vi "UnitTestSimulation.vi"(8 "error in (no error)":errorcluster) -> (0 "error out":errorcluster, 1 "LowerLimit":dbl[](array[numeric]), 2 "UpperLimit":dbl[](array[numeric]), 3 "Limit Testing":dbl[][](graph))   [LabVIEW 2021]
uses:
  <vilib>/measure/NI_MABase.lvlib
panel:
  in  "Signal":dbl[](array[numeric])=[1.1, 1.1, -0.9, -0.9, 1.1, 1.1, -0.9, -0.9, 1.1, 1.1, -0.9]
  out "Waveform":dbl[](array[numeric])
  in  "Upper Limit Y values":dbl[](array[numeric])=[1.1, 1.1, -0.9, -0.9, 1.1, 1.1, -0.9, -0.9, 1.1, 1.1, -0.9]
  in  "Lower Limit Y values":dbl[](array[numeric])=[0.9, 0.9, -1.1, -1.1, 0.9, 0.9, -1.1, -1.1, 0.9, 0.9, -1.1]
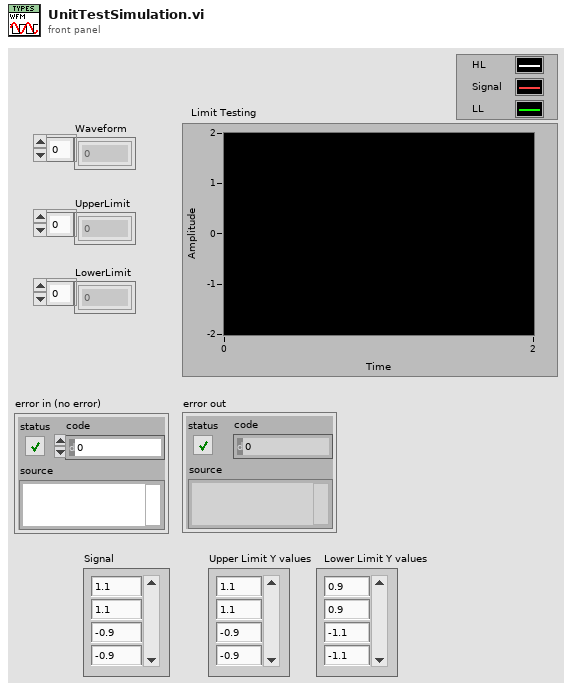
[diagram p1: front panel]
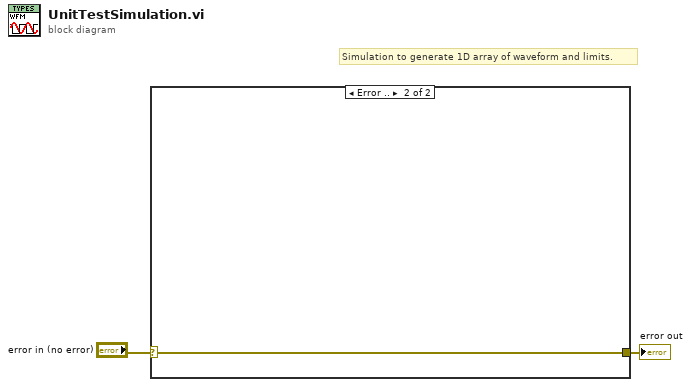
[diagram p0: block diagram]
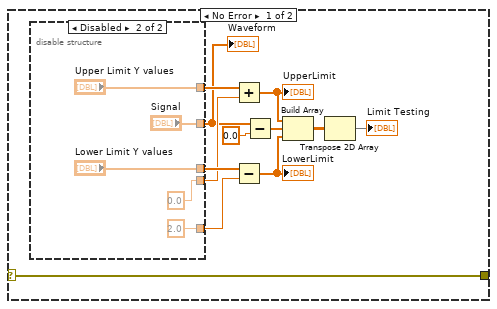
[diagram p2: hidden frame]
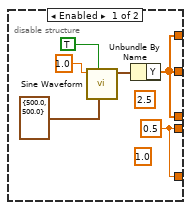
[diagram p3: hidden frame]
diagram:
  # "Simulation to generate 1D array of waveform and limits."
  n1 = case shown="Error .." "error in (no error)" {
    selector: "error in (no error)" -> [w3 w26]
    tunnel: [w3 w26] -> w1
    frame No Error {
      n2 = disable-structure shown="Disabled" {
        disable-tunnel: [w16 "Signal"] -> w6
        disable-tunnel: [w16 "Upper Limit Y values"] -> w10
        disable-tunnel: [w16 "Lower Limit Y values"] -> w9
        disable-tunnel: [w15 0.0] -> w8
        disable-tunnel: [w15 2.0] -> w7
        frame Enabled {
          (unwired) 1.0
          w15 = 0.5
          (unwired) 2.5 ("frequency")
          n3 = call <vilib>:"Sine Waveform.vi"("sampling info"=cluster{"Fs":dbl, "#s":dbl} {"Fs"=500.0, "#s"=500.0}, "reset signal"=TRUE, "frequency"=1.0) -> ("signal out"=w19:waveform(dbl))  [unwired: 7 in, 1 out]
          n4 = Unbundle By Name(w19) -> ("Y"=w16:dbl[])
        }
        frame Disabled {
        }
      }
      "Waveform" <- w6
      n5 = Add(x=w10, y=w8) -> (x+y=w5:dbl[])
      "UpperLimit" <- w5
      n6 = Subtract(x=w9, y=w7) -> (x-y=w4:dbl[])
      "LowerLimit" <- w4
      n7 = Subtract(x=w6, y=0.0) -> (x-y=w12:dbl[])
      n8 = Build Array(w5, w12, w4) -> (w14:dbl[][])
      n9 = Transpose 2D Array(2D array=w14) -> (transposed array=→"Limit Testing":dbl[][])
    }
    frame Error {
    }
  }
  "error out" <- w1
